vi "CombinedTrackingAndDistance(delete later NHB).vi"() -> ()   [LabVIEW 2011]
uses:
  <vilib>/Rock Robotics/SystemInterfaces/DIO/FPGA_DIOPWMChannel.ctl
  Vision/Servo Camera Example/Control States.ctl
  <vilib>/Rock Robotics/WPI/Camera/WPI_CameraWhite Balance Values.ctl
  <vilib>/Rock Robotics/WPI/Camera/WPI_CameraFrameRate.ctl
  <vilib>/Rock Robotics/WPI/Camera/WPI_CameraImageSize.ctl
  <vilib>/addons/control/pid/pid.llb/PID Control Input Filter (DBL).vi
  <vilib>/addons/control/pid/NI_PID_pid.lvlib
panel:
  in  "Enable servos":bool
  out "Distance (ft)":dbl
  in  "Servo Positions":cluster{"X":dbl, "Y":dbl}={"X"=85.52840986947938, "Y"=85.0} {"Y" scale=0.0..170.0; "X" scale=0.0..170.0}
  in  "Image Decimation":cluster{"X":dbl, "Y":dbl}={"X"=5.0, "Y"=4.0}
  out "Servo Tracking State 2":T2
  in  "Color Ranges":T3={"Hue"={"Min"=55, "Max"=93}, "Sat"={"Min"=41, "Max"=255}, "Luma"={"Min"=64, "Max"=255}}
  in  "Tracking Loop Sleep":u32=80
  in  "Servo Loop Sleep":u32=20
  in  "Smooth":bool=TRUE
  in  "Y Channel":T4=enum."PWM 2"
  in  "X Channel":T4
  in  "Camera IP Address":string="192.168.0.90"
  out "Processed Image":T5(plugin-control)
  out "Original Image":T5(plugin-control)
  in  "Annotate":bool=TRUE
  in  "Particle Count Limit":i32=10
  in  "Area Size Limit":i32=444
  in  "Score Limits":T6={"Rect Coverage"=76.0, "Aspect Ratio"=70.0, "X Edge Strength"=40.0, "Y Edge Strength"=60.0}
  in  "Camera Type":enum16{"206", "1011"}(ring)
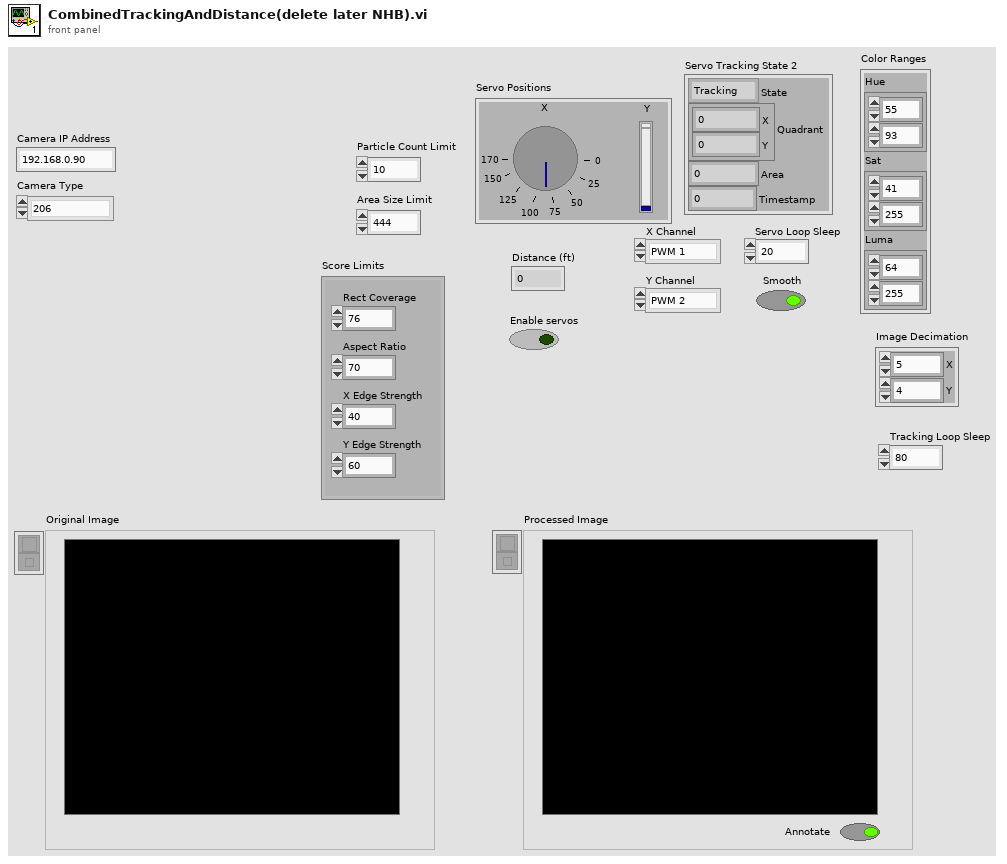
[diagram p1: front panel]
types:
  T1 = typedef "Control States.ctl" = enum16{"Tracking", "Lost Small", "Lost-Patience", "Search-Begin", "Searching", "Lost - Edge"}
  T2 = cluster{"State":T1, "Quadrant":cluster{"X":i32, "Y":i32}, "Area":i32, "Timestamp":u32}
  T3 = cluster{"Hue":cluster{"Min":i32, "Max":i32}, "Sat":cluster{"Min":i32, "Max":i32}, "Luma":cluster{"Min":i32, "Max":i32}}
  T4 = typedef "FPGA_DIOPWMChannel.ctl" = enum8{"PWM 1", "PWM 2", "PWM 3", "PWM 4", "PWM 5", "PWM 6", "PWM 7", "PWM 8", "PWM 9", "PWM 10", "Invalid"}
  T5 = typedef "IMAQ Image.ctl" = refnum<image>
  T6 = cluster{"Rect Coverage":dbl, "Aspect Ratio":dbl, "X Edge Strength":dbl, "Y Edge Strength":dbl}
  T7 = typedef "WPI_CameraImageSize.ctl" = enum16{"640x480", "320x240", "160x120"}
  T8 = typedef "WPI_CameraFrameRate.ctl" = u32
  T9 = typedef "WPI_CameraWhite Balance Values.ctl" = enum16{"Auto", "Fixed indoor", "Fixed outdoor 1", "Fixed outdoor 2", "Fixed fluorescent 1", "Fixed fluorescent 2", "Hold current"}
  T10 = typedef "WPI_CameraDevRef.ctl" = cluster{"Camera Address":string, "CameraStatus":errorcluster, "Acquire Image Notifier":refnum<notifier>}
  T11 = cluster{"Left":i32, "Top":i32, "Right":i32, "Bottom":i32}
  T12 = cluster{"State":T1, "Quadrant":cluster{"X":i32, "Y":i32}, "Area":i32, "millisecond timer value":u32}
  T13 = cluster{cluster{"Left":dbl, "Top":dbl, "Right":dbl, "Bottom":dbl}, dbl[]}[]
  T14 = cluster{"Left":dbl, "Top":dbl, "Right":dbl, "Bottom":dbl}
  T15 = typedef "WPI_ServoDeviceRef.ctl" = cluster{"DeviceStatus":errorcluster, "Digital Module":T16, "PWM Channel":T4, "DeadBand":T17}
  T16 = typedef "FPGA_TypedefDigitalModule.ctl" = enum16{"Digital Module 1", "Digital Module 2"}
  T17 = typedef "WPI_PWMDeadband.ctl" = cluster{"Name":string, "maxPositivePwm":i32, "minPositivePwm":i32, "centerPwm":i32, "maxNegativePwm":i32, "minNegativePwm":i32, "angularRange":u16}
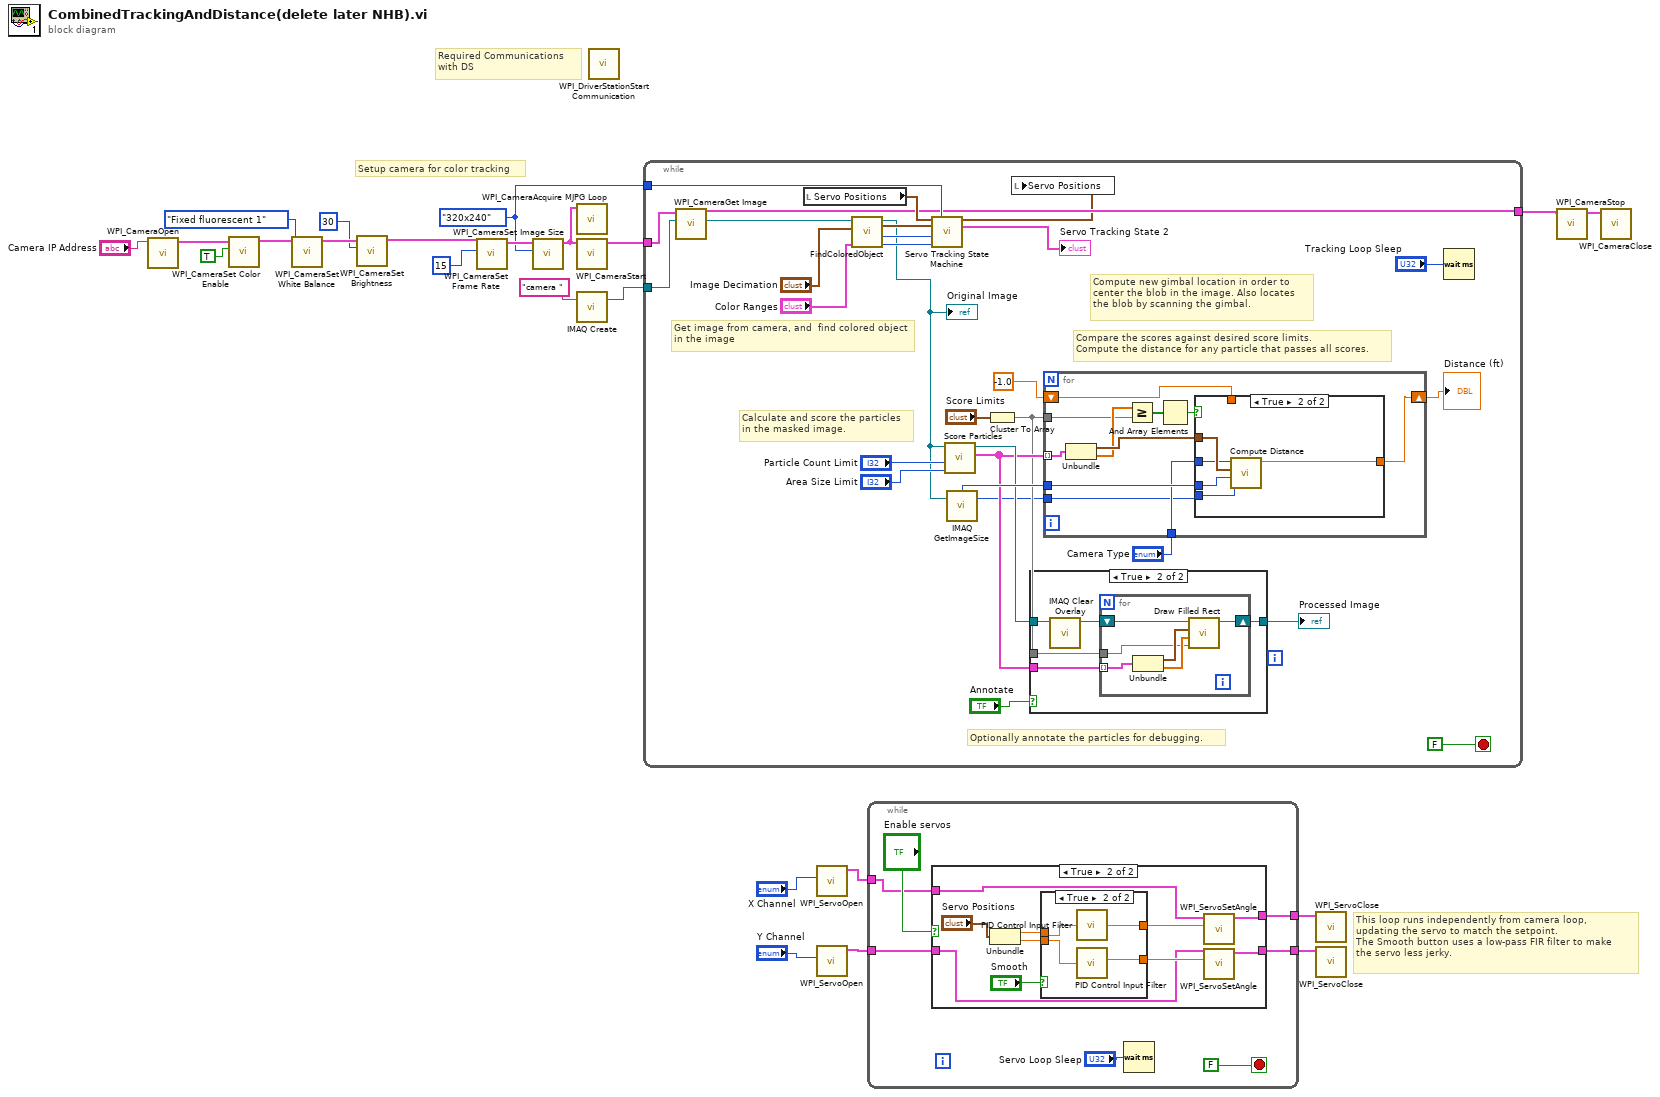
[diagram p0: block diagram]
diagram:
  w5 = WPI_CameraImageSize."320x240" ("Image Size")
  # "Required Communications\nwith DS"
  # "Setup camera for color tracking"
  # "This loop runs independently from camera loop,\nupdating the servo to match the setpoint.\nThe Smooth button uses a low-pass FIR filter to make\nthe servo less jerky."
  n1 = call <vilib>:"WPI_CameraOpen.vi"("Camera Address"="Camera IP Address") -> ("CameraDevRef"=w2:T10)  [unwired: 9 in, 1 out]
  n2 = call <vilib>:"WPI_CameraSet Color Enable.vi"("Color Enabled"=TRUE, "CameraDevRef"=w2) -> ("CameraDevRef Out"=w21:T10)  [unwired: 8 in, 1 out]
  n3 = call <vilib>:"WPI_CameraSet White Balance.vi"("White Balance"=WPI_CameraWhite_Balance_Values."Fixed fluorescent 1", "CameraDevRef"=w21) -> ("CameraDevRef Out"=w19:T10)  [unwired: 8 in, 1 out]
  n4 = call <vilib>:"WPI_CameraSet Brightness.vi"("Brightness"=30, "CameraDevRef"=w19) -> ("CameraDevRef Out"=w1:T10)  [unwired: 8 in, 1 out]
  n5 = call <vilib>:"WPI_CameraSet Frame Rate.vi"("Frame Rate (fps)"=T8 15, "CameraDevRef"=w1) -> ("CameraDevRef Out"=w9:T10)  [unwired: 1 in, 8 out]
  n6 = call <vilib>:"WPI_CameraSet Image Size.vi"("Image Size"=w5, "CameraDevRef"=w9) -> ("CameraDevRef Out"=w8:T10)  [unwired: 1 in, 8 out]
  n7 = call <vilib>:"WPI_CameraAcquire MJPG Loop.vi"("CameraDevRef"=w8) -> ()  [unwired: 11 in]
  n8 = call <vilib>:"WPI_CameraStart.vi"("CameraDevRef"=w8) -> ("CameraDevRef Out"=w7:T10)  [unwired: 1 in, 9 out]
  n9 = call "IMAQ Create"("Image Name"="camera ") -> ("New Image"=w6:T5)  [unwired: 3 in, 2 out]
  n10 = call <vilib>:"WPI_DriverStationStart Communication.vi"() -> ()  [unwired: 1 in, 11 out]
  n11 = while {
    tunnel: w7 -> [w41]
    tunnel: w6 -> [w40]
    tunnel: w5 -> [w30]
    tunnel: [w29] -> w3
    stop <- FALSE stop-if-true
    # "Compute new gimbal location in order to\ncenter the blob in the image. Also locates\nthe blob by scanning the gimbal."
    # "Get image from camera, and  find colored object in the image"
    # "Optionally annotate the particles for debugging."
    # "Compare the scores against desired score limits.\nCompute the distance for any particle that passes all scores."
    # "Calculate and score the particles\nin the masked image."
    n12 = call <vilib>:"WPI_CameraGet Image.vi"("Image"=w40, "CameraDevRef"=w41) -> ("Image Out"=w31:T5, "CameraDevRef Out"=w29:T10)  [unwired: 1 in, 7 out]
    n13 = local read "Servo Positions"() -> (w36:cluster{"X":dbl, "Y":dbl})
    n14 = call "FindColoredObject.vi"("Color Range"="Color Ranges", "Decimate by"="Image Decimation", "Color Image In"=w31) -> ("Area"=w32:i32, "Particles"=w34:i32, "Rectangle"=w35:T11, "Mask Image"=w24:T5)  [unwired: 3 out]
    "Original Image" <- w24
    n15 = call "Servo Tracking State Machine.vi"("Servo Positions In"=w36, "Image Size"=w30, "Rectangle"=w35, "Particles"=w34, "Area"=w32) -> ("Servo Positions"=w28:cluster{"X":dbl, "Y":dbl}, "Tracking State Info"=→"Servo Tracking State 2":T12)  [unwired: 2 in, 7 out]
    n16 = call "Score Particles.vi"("Area Size Limit"="Area Size Limit", "Particle Count Limit"="Particle Count Limit", "Image Refnum in"=w24) -> ("Scored Particle Info"=w47:T13, "Image Refnum out"=w51:T5)  [unwired: 7 in]
    n17 = call "IMAQ GetImageSize"("Image"=w24) -> ("Y Resolution"=w42:i32, "X Resolution"=w52:i32)  [unwired: 3 in, 1 out]
    n18 = Cluster To Array(cluster="Score Limits") -> (array=w45:dbl[])
    n19 = local write "Servo Positions"(w28) -> ()
    n20 = case shown="True" "Annotate" {
      tunnel: w51 -> [w53 w58]
      tunnel: [w53 w57] -> w48
      tunnel: w47 -> [_ w55]
      tunnel: w45 -> [_ w54]
      frame False {
      }
      frame True {
        n21 = call "IMAQ Clear Overlay"("Image"=w58) -> ("Image Out"=w56:T5)  [unwired: 2 in, 8 out]
        n22 = for {
          shift-right: [w63] -> w57
          shift-left: w56 -> [w64]
          tunnel: w55 -> [w60] mode=indexing
          tunnel: w54 -> [w59]
          n23 = Unbundle(w60) -> (w61:T14, w62:dbl[])
          n24 = call "Draw Filled Rect.vi"("Limits"=w59, "Scores"=w62, "Bounding Box"=w61, "image in"=w64) -> ("image out"=w63:T5)  [unwired: 7 in]
        }
      }
    }
    "Processed Image" <- w48
    n25 = for {
      shift-right: [w66] -> w27
      shift-left: -1.0 ("Distance (ft)") -> [w65]
      tunnel: w52 -> [w75]
      tunnel: w47 -> [w73] mode=indexing
      tunnel: w45 -> [w68]
      tunnel: "Camera Type" -> [w72]
      tunnel: w42 -> [w67]
      n26 = Unbundle(w73) -> (w74:T14, w69:dbl[])
      n27 = Greater Or Equal?(x=w69, y=w68) -> (x >= y?=w71:bool[])
      n28 = And Array Elements(Boolean array=w71) -> (logical AND=w70:bool)
      n29 = case shown="True" w70 {
        tunnel: w74 -> [_ w80]
        tunnel: w75 -> [_ w81]
        tunnel: w72 -> [_ w79]
        tunnel: w67 -> [_ w78]
        tunnel: [w76 w77] -> w66
        tunnel: w65 -> [w76 _]
        frame False {
          # "Use the value from the\nother box-targets"
          # "This distance is not\nwithin range"
        }
        frame True {
          n30 = call "Compute Distance.vi"("Y Image Resolution"=w78, "X Image Resolution"=w81, "Bounding Box"=w80, "Camera Type"=w79) -> ("Distance (ft)"=w77:dbl)  [unwired: 6 in, 1 out]
        }
      }
    }
    "Distance (ft)" <- w27
    n31 = Wait (ms)(milliseconds to wait="Tracking Loop Sleep") -> ()  [unwired: 1 out]
  }
  n32 = call <vilib>:"WPI_ServoOpen.vi"("PWM Channel"="X Channel") -> ("ServoDeviceRef"=w15:T15)  [unwired: 3 in, 7 out]
  n33 = call <vilib>:"WPI_ServoOpen.vi"("PWM Channel"="Y Channel") -> ("ServoDeviceRef"=w14:T15)  [unwired: 3 in, 7 out]
  n34 = while {
    tunnel: w15 -> [w84]
    tunnel: [w88] -> w13
    tunnel: w14 -> [w83]
    tunnel: [w86] -> w12
    stop <- FALSE stop-if-true
    n35 = case shown="True" "Enable servos" {
      tunnel: [w90 w100] -> w88
      tunnel: [w89 w99] -> w86
      tunnel: w84 -> [w90 w92]
      tunnel: w83 -> [w89 w91]
      frame False {
        # "Do not run the servos"
      }
      frame True {
        n36 = Unbundle("Servo Positions") -> ("X"=w98:dbl, "Y"=w96:dbl)
        n37 = case shown="True" "Smooth" {
          tunnel: w98 -> [w102 w106]
          tunnel: [w102 w105] -> w97
          tunnel: w96 -> [w101 w104]
          tunnel: [w101 w103] -> w95
          frame False {
          }
          frame True {
            n38 = call-poly <vilib>:"PID Control Input Filter.vi"("input"=w106) -> ("output"=w105:dbl)  [unwired: 1 in, 3 out]
            n39 = call-poly <vilib>:"PID Control Input Filter.vi"("input"=w104) -> ("output"=w103:dbl)  [unwired: 1 in, 3 out]
          }
        }
        n40 = call <vilib>:"WPI_ServoSetAngle.vi"("Angle"=w97, "ServoDeviceRef"=w92) -> ("ServoDeviceRef"=w100:T15)  [unwired: 1 in, 8 out]
        n41 = call <vilib>:"WPI_ServoSetAngle.vi"("Angle"=w95, "ServoDeviceRef"=w91) -> ("ServoDeviceRef"=w99:T15)  [unwired: 1 in, 8 out]
      }
    }
    n42 = Wait (ms)(milliseconds to wait="Servo Loop Sleep") -> ()  [unwired: 1 out]
  }
  n43 = call <vilib>:"WPI_ServoClose.vi"("MotorControlDevRef"=w13) -> ()  [unwired: 1 in, 10 out]
  n44 = call <vilib>:"WPI_ServoClose.vi"("MotorControlDevRef"=w12) -> ()  [unwired: 1 in, 10 out]
  n45 = call <vilib>:"WPI_CameraStop.vi"("CameraDevRef"=w3) -> ("CameraDevRef Out"=w4:T10)  [unwired: 1 in, 9 out]
  n46 = call <vilib>:"WPI_CameraClose.vi"("CameraDevRef"=w4) -> ()  [unwired: 1 in, 10 out]
